vi "stage_close.vi"(8 "error in (no error)":errorcluster, 11 "Stage reference":T1) -> ()   [LabVIEW 2018]
uses:
  stage_reference_type.ctl
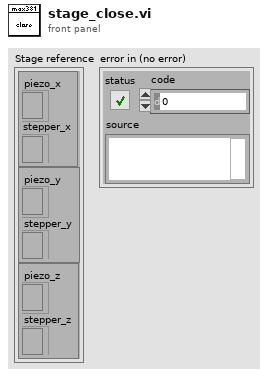
[diagram p1: front panel]
types:
  T1 = typedef "stage_reference_type.ctl" = cluster{cluster{"piezo_x":refnum<k7>, "stepper_x":refnum<k7>}, cluster{"piezo_y":refnum<k7>, "stepper_y":refnum<k7>}, cluster{"piezo_z":refnum<k7>, "stepper_z":refnum<k7>}}
  T2 = cluster{"piezo_x":refnum<k7>, "stepper_x":refnum<k7>}
  T3 = cluster{"piezo_y":refnum<k7>, "stepper_y":refnum<k7>}
  T4 = cluster{"piezo_z":refnum<k7>, "stepper_z":refnum<k7>}
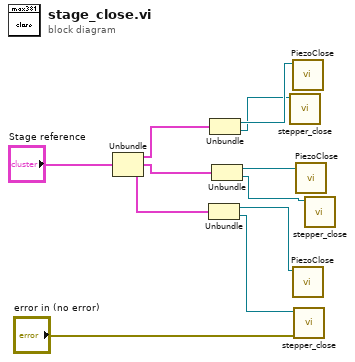
[diagram p0: block diagram]
diagram:
  n1 = Unbundle("Stage reference") -> (w10:T2, w9:T3, w8:T4)
  n2 = Unbundle(w8) -> ("piezo_z"=w5:refnum<k7>, "stepper_z"=w3:refnum<k7>)
  n3 = Unbundle(w10) -> ("piezo_x"=w7:refnum<k7>, "stepper_x"=w2:refnum<k7>)
  n4 = Unbundle(w9) -> ("piezo_y"=w6:refnum<k7>, "stepper_y"=w4:refnum<k7>)
  n5 = call <userlib>:"stepper_close.vi"("reference"=w2) -> ()  [unwired: 9 in, 2 out]
  n6 = call <userlib>:"PiezoClose.vi"("reference"=w7) -> ()  [unwired: 5 in, 2 out]
  n7 = call <userlib>:"PiezoClose.vi"("reference"=w5) -> ()  [unwired: 5 in, 2 out]
  n8 = call <userlib>:"stepper_close.vi"("error in (no error)"="error in (no error)", "reference"=w3) -> ()  [unwired: 8 in, 2 out]
  n9 = call <userlib>:"PiezoClose.vi"("reference"=w6) -> ()  [unwired: 5 in, 2 out]
  n10 = call <userlib>:"stepper_close.vi"("reference"=w4) -> ()  [unwired: 9 in, 2 out]
